vi "Field_C evaluate status.vi"(2 "PSU Status in":T8 {"Trip Current" format="%.3f"; "Trip Field" format="%.4f"; "Voltage" format="%.2f"; "Field Constant" format="%.6f"; "MID Setpoint (T)" format="%.4f"; "MID Setpoint (A)" format="%.3f"; "MAX Setpoint (T)" format="%.4f"; "MAX Setpoint (A)" format="%.3f"; "Heater Voltage" format="%.2f"; "V Limit (V)" format="%.2f"; "Ramp Rate (A/s)" format="%.3f"; "Output (A)" format="%.3f"; "Output (T)" format="%.4f"; "Persistent Current" format="%.3f"; "Persistent Field" format="%.4f"}, 4 "Overall status in":T1, 5 "Magnet Constants":T7={"Switch resistant [K]"=5.0, "Switch superconducting [K]"=4.0, "First stage critical temperature [K]"=50.0, "Second stage critical temperature [K]"=5.0, "Inner magnet critical temperature [K]"=6.0, "Outer magnet critical temperature [K]"=5.0, "Field Constant [T/A]"=0.14911, "Maximum Current [A]"=107.3, "Maximum field [T]"=16.0, "Maximum source ramp [A/s]"=0.5, "Source precision [T]"=2e-05, "Ramp limits [A/s]"=[0.0506, 0.038, 0.0285, 0.0213, 0.0104], "Field limits [T]"=[3.0, 9.6, 13.3, 15.5, 16.0], "SMS"="COM3", "LSC218"="COM1"}) -> (0 "Overall status out":T1)   [LabVIEW 2024, in "Magnet module.lvlib"]
doc: "Evaluates actual overall status of the magnet module.\nResult should be send as a message to master module."
uses:
  Magnet module.lvlib
  <instrlib>/SMS drivers/Public/PSU Status.ctl
  ctl/Overall status.ctl
  ctl/SetField data.ctl
  ctl/Magnet mode public.ctl
  ctl/Actual magnet state.ctl
  ctl/Magnet mode.ctl
  ctl/RampingOutput.ctl
  ctl/Magnet config constants.ctl
  <instrlib>/SMS drivers/Cryogenic Ltd SMSXXX.lvlib
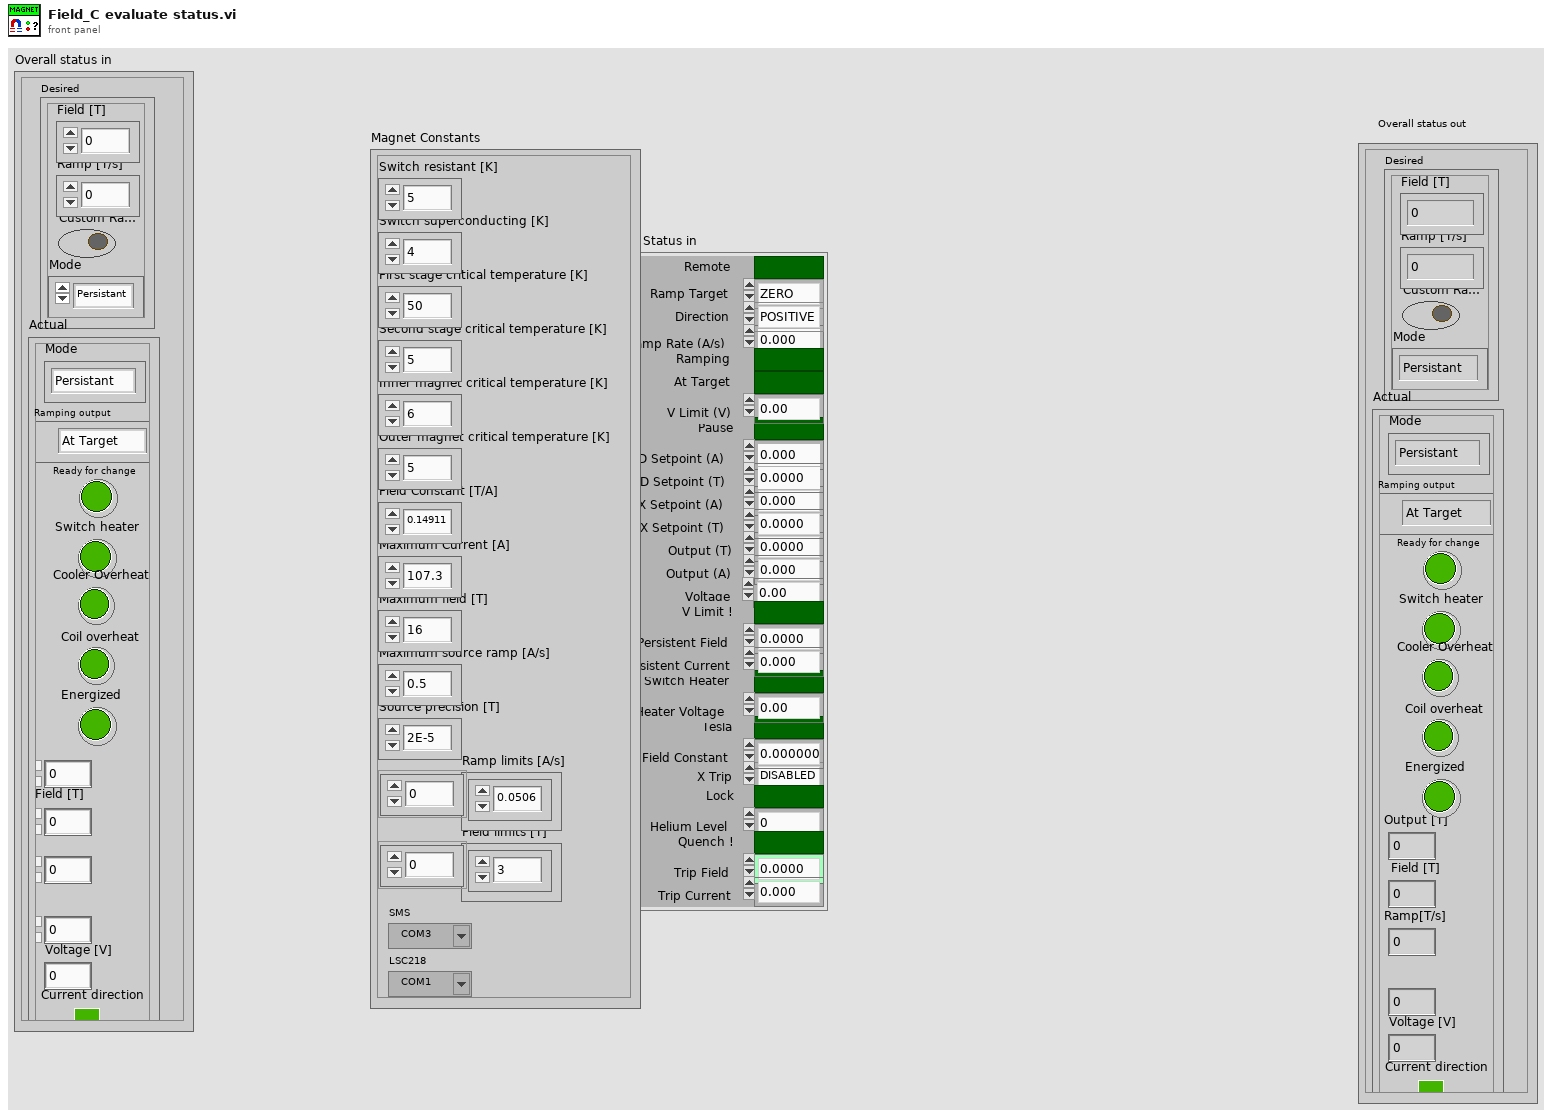
[diagram p1: front panel]
types:
  T1 = typedef "Magnet module.lvlib/Overall status.ctl" = cluster{"Desired":T2, "Actual":T4}
  T2 = typedef "Magnet module.lvlib/SetField data.ctl" = cluster{"Field [T]":dbl, "Ramp [T/s]":dbl, "Custom Ramp?":bool, "Mode":T3}
  T3 = typedef "Magnet module.lvlib/Magnet mode public.ctl" = enum16{"Persistant", "Ramping"}
  T4 = typedef "Magnet module.lvlib/Actual magnet state.ctl" = cluster{"Mode":T5, "Ramping output":T6, "Ready for change":bool, "Switch heater":bool, "Cooler Overheat":bool, "Coil overheat":bool, "Energized":bool, "Output [T]":dbl, "Field [T]":dbl, "Ramp[T/s]":dbl, "Switch\ntemperature [K]":dbl, "Voltage [V]":dbl, "Current direction":bool}
  T5 = typedef "Magnet module.lvlib/Magnet mode.ctl" = enum16{"Persistant", "Switching", "Ramping", "Quenched"}
  T6 = typedef "Magnet module.lvlib/RampingOutput.ctl" = enum16{"At Target", "Go up", "Go down"}
  T7 = typedef "Magnet module.lvlib/Magnet config constants.ctl" = cluster{"Switch resistant [K]":dbl, "Switch superconducting [K]":dbl, "First stage critical temperature [K]":dbl, "Second stage critical temperature [K]":dbl, "Inner magnet critical temperature [K]":dbl, "Outer magnet critical temperature [K]":dbl, "Field Constant [T/A]":dbl, "Maximum Current [A]":dbl, "Maximum field [T]":dbl, "Maximum source ramp [A/s]":dbl, "Source precision [T]":dbl, "Ramp limits [A/s]":dbl[], "Field limits [T]":dbl[], "SMS":refnum<visa-resource-name>, "LSC218":refnum<visa-resource-name>}
  T8 = typedef "Cryogenic Ltd SMSXXX.lvlib/PSU Status.ctl" = cluster{"Ramp Target":enum16{"ZERO", "MID", "MAX"}, "Pause":bool, "Switch Heater":bool, "Persistent Field":dbl, "Persistent Current":dbl, "Tesla":bool, "Output (T)":dbl, "Output (A)":dbl, "X Trip":enum16{"DISABLED", "ENABLED", "ACTIVE"}, "Ramp Rate (A/s)":dbl, "V Limit (V)":dbl, "Heater Voltage":dbl, "MAX Setpoint (A)":dbl, "MAX Setpoint (T)":dbl, "MID Setpoint (A)":dbl, "MID Setpoint (T)":dbl, "Lock":bool, "Field Constant":dbl, "Remote":bool, "Direction":enum16{"POSITIVE", "NEGATIVE", "OPEN", "UNIPOLAR"}, "Helium Level":u16, "Quench !":bool, "Voltage":dbl, "V Limit !":bool, "Ramping":bool, "At Target":bool, "Trip Field":dbl, "Trip Current":dbl}
  T9 = enum16{"POSITIVE", "NEGATIVE", "OPEN", "UNIPOLAR"}
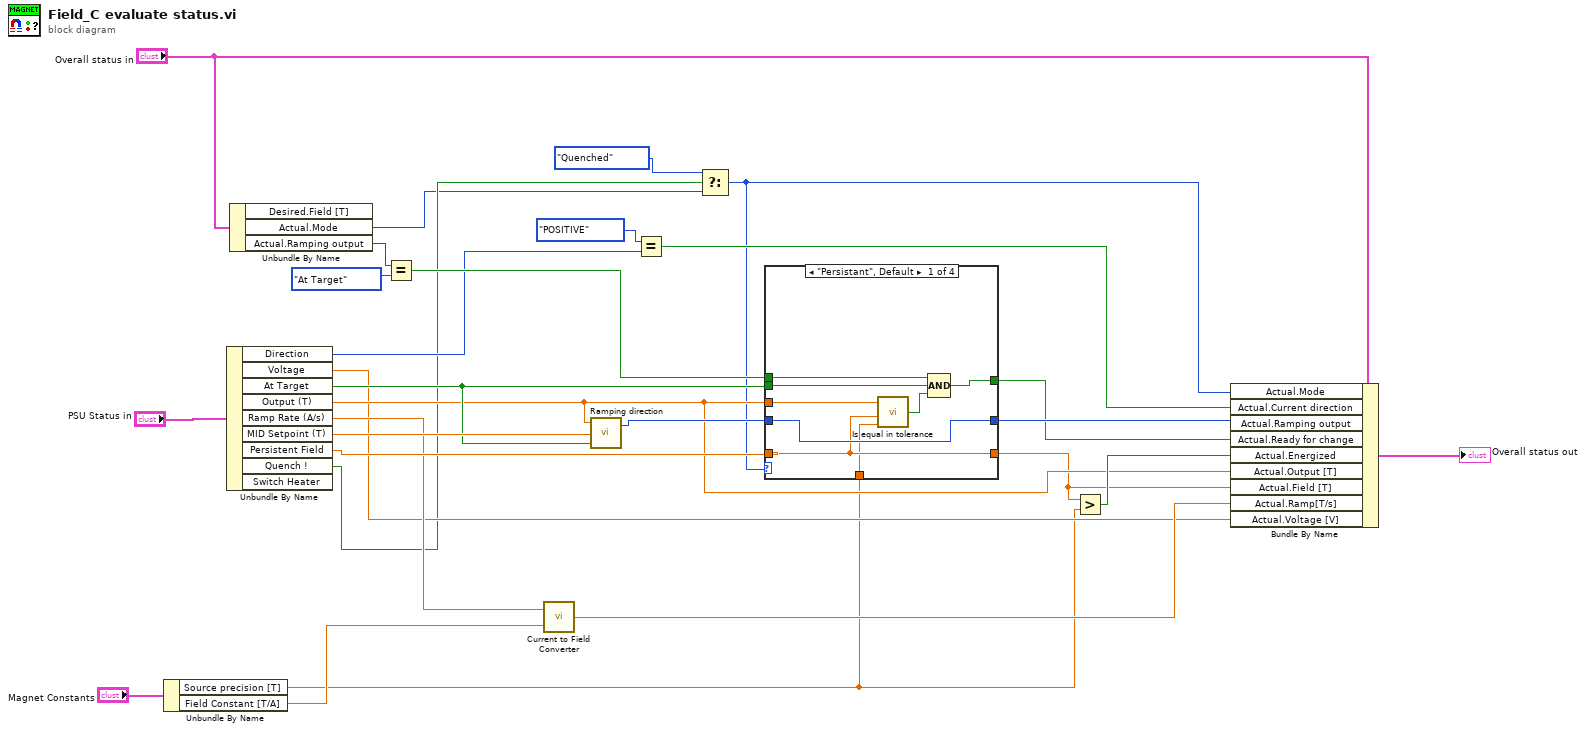
[diagram p0: block diagram]
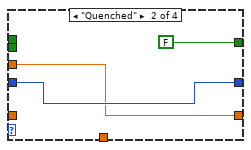
[diagram p2: hidden frame]
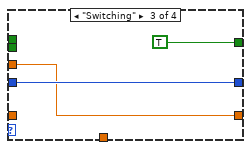
[diagram p3: hidden frame]
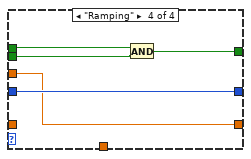
[diagram p4: hidden frame]
diagram:
  n1 = Unbundle By Name("Magnet Constants") -> ("Source precision [T]"=w3:dbl, "Field Constant [T/A]"=w22:dbl)
  n2 = Unbundle By Name("PSU Status in") -> ("Direction"=w14:T9, "Voltage"=w7:dbl, "At Target"=w27:bool, "Output (T)"=w10:dbl, "Ramp Rate (A/s)"=w21:dbl, "MID Setpoint (T)"=w28:dbl, "Persistent Field"=w24:dbl, "Quench !"=w6:bool)  [unwired: 1 out]
  n3 = Unbundle By Name("Overall status in") -> ("Actual.Mode"=w2:T5, "Actual.Ramping output"=w17:T6)  [unwired: 1 out]
  n4 = Equal?(x=w17, y=RampingOutput."At Target" ("Actual.Ramping output")) -> (x = y?=w15:bool)
  n5 = call "Current to Field Converter.vi"("Field constant [T/A]"=w22, "Current in [A]"=w21) -> ("Field out [T]"=w8:dbl)
  n6 = call "Ramping direction.vi"("At target"=w27, "Actual targget [T]"=w28, "Actual output [T]"=w10) -> ("Ramping direction"=w25:T6)  [unwired: 1 in]
  n7 = Equal?(x=T9."POSITIVE" ("Direction"), y=w14) -> (x = y?=w4:bool)
  n8 = Select(t=Magnet_mode."Quenched" ("Actual.Mode"), s=w6, f=w2) -> (s? t:f=w1:T5)
  n9 = case shown="\"Persistant\", Default" w1 {
    tunnel: [w36 FALSE ("Is stabe") TRUE ("Ready") w43] -> w12
    tunnel: w24 -> [w33 _ _ _]
    tunnel: w10 -> [w34 w38 w40 w46]
    tunnel: w25 -> [w35 w39 w42 w47]
    tunnel: [w35 w39 w42 w47] -> w13
    tunnel: w27 -> [w30 _ _ w45]
    tunnel: [w33 w38 w40 w46] -> w9
    tunnel: w15 -> [w31 _ _ w44]
    tunnel: w3 -> [w29 _ _ _]
    frame "Persistant", Default {
      n10 = call "Is equal in tolerance.vi"("Absolut tolerance"=w29, "Reference value"=w33, "Input value"=w34) -> ("Is in range"=w32:bool)  [unwired: 1 in]
      n11 = Compound Arithmetic op=AND(w31, w30, w32) -> (w36:bool)
    }
    frame "Quenched" {
    }
    frame "Switching" {
    }
    frame "Ramping" {
      n12 = And(x=w44, y=w45) -> (x .and. y?=w43:bool)
    }
  }
  n13 = Greater?(x=w9, y=w3) -> (0:w11:bool)
  n14 = Bundle By Name(cluster="Overall status in", "Actual.Mode"=w1, "Actual.Current direction"=w4, "Actual.Ramping output"=w13, "Actual.Ready for change"=w12, "Actual.Energized"=w11, "Actual.Output [T]"=w10, "Actual.Field [T]"=w9, "Actual.Ramp[T/s]"=w8, "Actual.Voltage [V]"=w7) -> (→"Overall status out":T1)
